vi "PXIe-6592-IP-Node.vi"() -> ()   [LabVIEW 2017]
uses:
  <vilib>/Platform/TimedLoop/XDataNode/timing_clust.ctl
  <vilib>/Platform/TimedLoop/XDataNode/nitl_modes.ctl
  <vilib>/Platform/TimedLoop/XDataNode/wakeup.ctl
  <vilib>/rvi/IPIntegrationNode/IPINode_Typedef/niFpgaIPINodeSupportedFamilies.ctl
  <vilib>/rvi/Emulation/niFpgaSctlEmulationGetInTimedLoop.vi
  <vilib>/rvi/Emulation/niFpgaEmulationReportErrorSimple.vi
  <vilib>/rvi/Emulation/niFpgaGetClockAttributes.vi
  <vilib>/rvi/Emulation/niFpgaCriticalErrorInLSC.vi
  <vilib>/rvi/interface/RandomDataEmulation/niFpgaRandomDataHandleErrors.vi
  <vilib>/rvi/IPIntegrationNode/IPINode_Utilities/niFpgaIPINodeSimCore.vi
  <vilib>/Platform/TimedLoop/XDataNode/XDataNode.xnode
  <vilib>/rvi/DataTransferAndStorage/Container/XNode/niFpgaContainer.xnode
  <vilib>/rvi/interface/RandomDataEmulation/nirviRandomDataFpgaReadWriteTemplate.vi
  <vilib>/rvi/IPIntegrationNode/IPINode_Xnode/niFpgaIPINode.xnode
  LabVIEW-Customer-IP-Node/Customer_Provided_Code/IP_BlockSimFiles/xsim.dir/wrapper_for_labview/xsimk4481C290FC144DB4A5E15DBB3E2EEBFF.dll
  <vilib>/Platform/TimedLoop/XDataNode/XDNodeRunTimeDep.lvlib
panel:
  in  "control_i\\rstn":bool
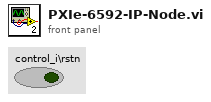
[diagram p1: front panel]
types:
  T1 = typedef "XDNodeRunTimeDep.lvlib/timing_clust.ctl" = cluster{"Expected End [f-1]":u64, "Actual End [f-1]":u64, "Finished Late? [f-1]":bool, "Expected End [i-1]":u64, "Actual End [i-1]":u64, "Finished Late? [i-1]":bool, "Expected Start [i]":u64, "Actual Start [i]":u64, "Expected Start [f]":u64, "Actual Start [f]":u64, "Source Name":string, "Structure Name":string, "Period":i64, "Deadline":i64, "Offset":i64, "Start":i64, "Priority":i32, "Timeout":i32, "Mode":T2, "Wakeup Reason":T3, "Error":errorcluster, "Source Type":string, "Secondary Source Type":string, "Global End Time":u64, "Global Start Time":u64, "Frame Duration":u64, "Iteration Duration":u64, "Assigned CPU":i32, "I/O Scan Engine Mode":u32}
  T2 = typedef "XDNodeRunTimeDep.lvlib/nitl_modes.ctl" = enum32{"No Change", "Process missed periods, maintain original phase", "Discard missed periods, maintain original phase", "Process missed periods, ignore original phase", "Discard missed periods, ignore original phase"}
  T3 = typedef "XDNodeRunTimeDep.lvlib/wakeup.ctl" = enum32{"Normal", "Aborted", "Asynchronous wakeup", "Timing source error", "Timed loop error", "Timeout"}
  T4 = typedef "niFpgaIPINodeSupportedFamilies.ctl" = cluster{"unlimited?":bool, "supported targets":string[]}
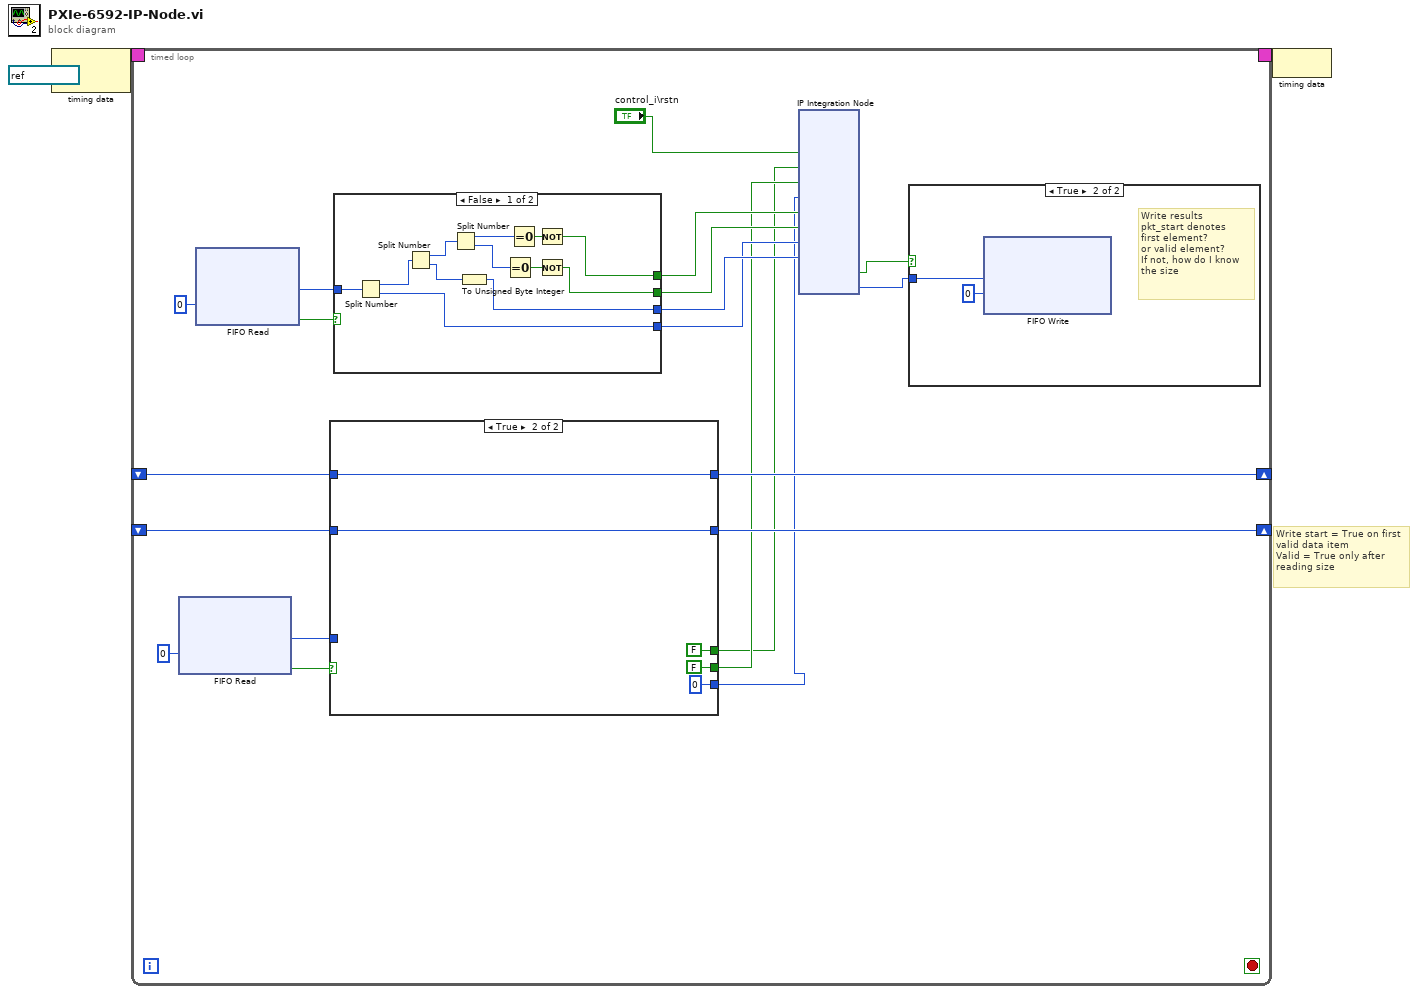
[diagram p0: block diagram]
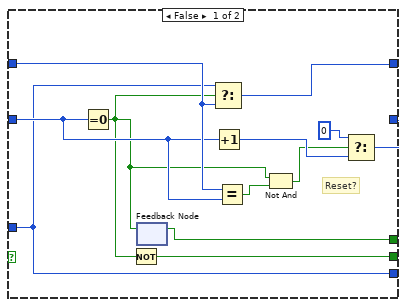
[diagram p3: hidden frame]
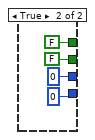
[diagram p4: hidden frame]
diagram:
  # "Write start = True on first\nvalid data item\nValid = True only after\nreading size"
  n1 = node-c288(refnum<k21> "125MHz" ("Source Name")) -> (w3:T1)
  n2 = timed-loop {
    timing: w3 -> [_]
    timing-out: [_] -> w2
    shift-right: [w16] -> _
    shift-left: _ -> [w17]
    shift-right: [w15] -> _
    shift-left: _ -> [w18]
    stop <- _ stop-if-true
    n3 = xnode ("FIFO Read")("Timeout"=0) -> ("Element"=w14:u64, "Timed Out?"=w19:bool)  [unwired: 1 in, 1 out]
    n4 = xnode ("FIFO Read")("Timeout"=0) -> ("Element"=w21:u64, "Timed Out?"=w22:bool)  [unwired: 1 in, 1 out]
    n5 = case shown="True" w19 {
      tunnel: w17 -> [w109 w115]
      tunnel: w18 -> [w108 w114]
      tunnel: [w110 w115] -> w16
      tunnel: [w105 w114] -> w15
      tunnel: w14 -> [w99 _]
      tunnel: [w101 FALSE] -> w6
      tunnel: [w100 FALSE] -> w7
      tunnel: [w99 u64 0 ("Element")] -> w8
      frame False {
        # "Reset?"
        n6 = Equal To 0?(x=w108) -> (x = 0?=w102:bool)
        n7 = Not(x=w102) -> (.not. x?=w100:bool)
        n8 = feedback-in #1(w102) -> ()
        n9 = feedback #1() -> (w101:bool)  [unwired: 1 in]
        n10 = Select(t=w99, s=w102, f=w109) -> (s? t:f=w110:u64)
        n11 = Increment(x=w108) -> (x+1=w107:i16)
        n12 = Equal?(x=w109, y=w108) -> (x = y?=w104:bool)
        n13 = Not And(1:w104, 2:w102) -> (0:w103:bool)
        n14 = Select(t=i16 0, s=w103, f=w107) -> (s? t:f=w105:i16)
      }
      frame True {
      }
    }
    n15 = case shown="False" w22 {
      tunnel: w21 -> [w127 _]
      tunnel: [w119 FALSE] -> w12
      tunnel: [w118 FALSE] -> w11
      tunnel: [w117 u8 0] -> w10
      tunnel: [w116 u32 0] -> w9
      frame False {
        n16 = Split Number(x=w127) -> (hi(x)=w126:u32, lo(x)=w116:u32)
        n17 = Split Number(x=w126) -> (hi(x)=w124:u16, lo(x)=w125:u16)
        n18 = Split Number(x=w124) -> (hi(x)=w123:u8, lo(x)=w122:u8)
        n19 = To Unsigned Byte Integer(number=w125) -> (unsigned 8bit integer=w117:u8)
        n20 = Equal To 0?(x=w122) -> (x = 0?=w120:bool)
        n21 = Equal To 0?(x=w123) -> (x = 0?=w121:bool)
        n22 = Not(x=w121) -> (.not. x?=w119:bool)
        n23 = Not(x=w120) -> (.not. x?=w118:bool)
      }
      frame True {
      }
    }
    n24 = xnode "IP Integration Node"("rstn"="control_i\\rstn", "start"=w6, "valid"=w7, "data"=w8, "cfg_start"=w12, "cfg_valid"=w11, "cfg_data"=w9, "cfg_addr"=w10) -> ("pkt_start"=w5:bool, "pkt_out"=w4:u64)  [unwired: 2 in]
    n25 = case shown="True" w5 {
      tunnel: w4 -> [_ w98]
      frame False {
      }
      frame True {
        # "Write results\npkt_start denotes\nfirst element?\nor valid element?\nIf not, how do I know\nthe size"
        n26 = xnode ("FIFO Write")("Element"=w98, "Timeout"=0) -> ()  [unwired: 1 in, 2 out]
      }
    }
  }
  n27 = node-c288(w2) -> ()
